vi "test_resist_new.vi"() -> ()   [LabVIEW 2015]
panel:
  out "String":string
  in  "Stop Button":bool
  in  "Open Button":bool
  out "Waveform Chart":dbl(graph)
  out "Voltage value":string
  in  "Refresh Button":bool
  in  "Close VI":bool
  in  "Run Test":bool
  out "error out":errorcluster[](array[cluster])
  in  "Measure time (s)":string="300"
  in  "Acquisition frequency (s)":string="1"
  in  "Precision":string="3"
  # "Insert measure parameters and then click \"Run test\""
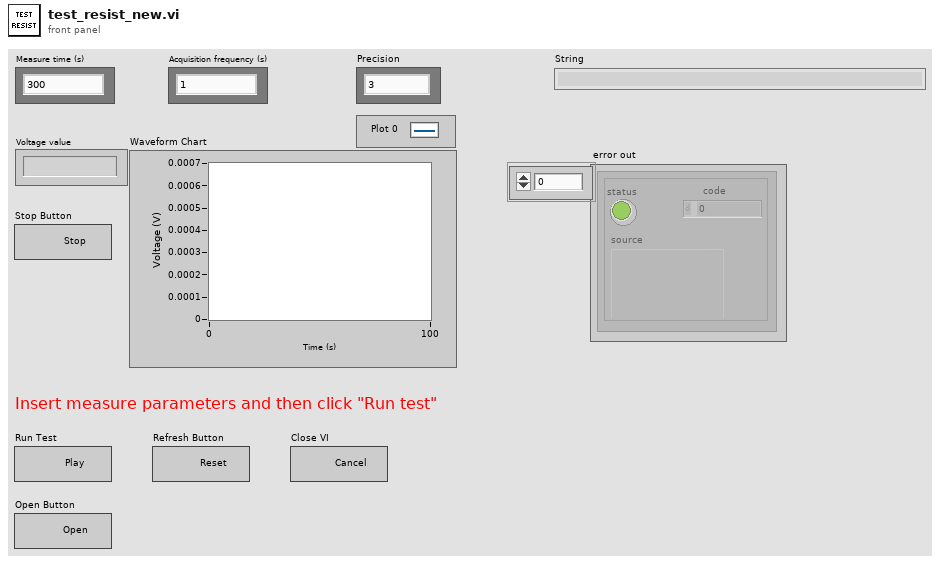
[diagram p1: front panel]
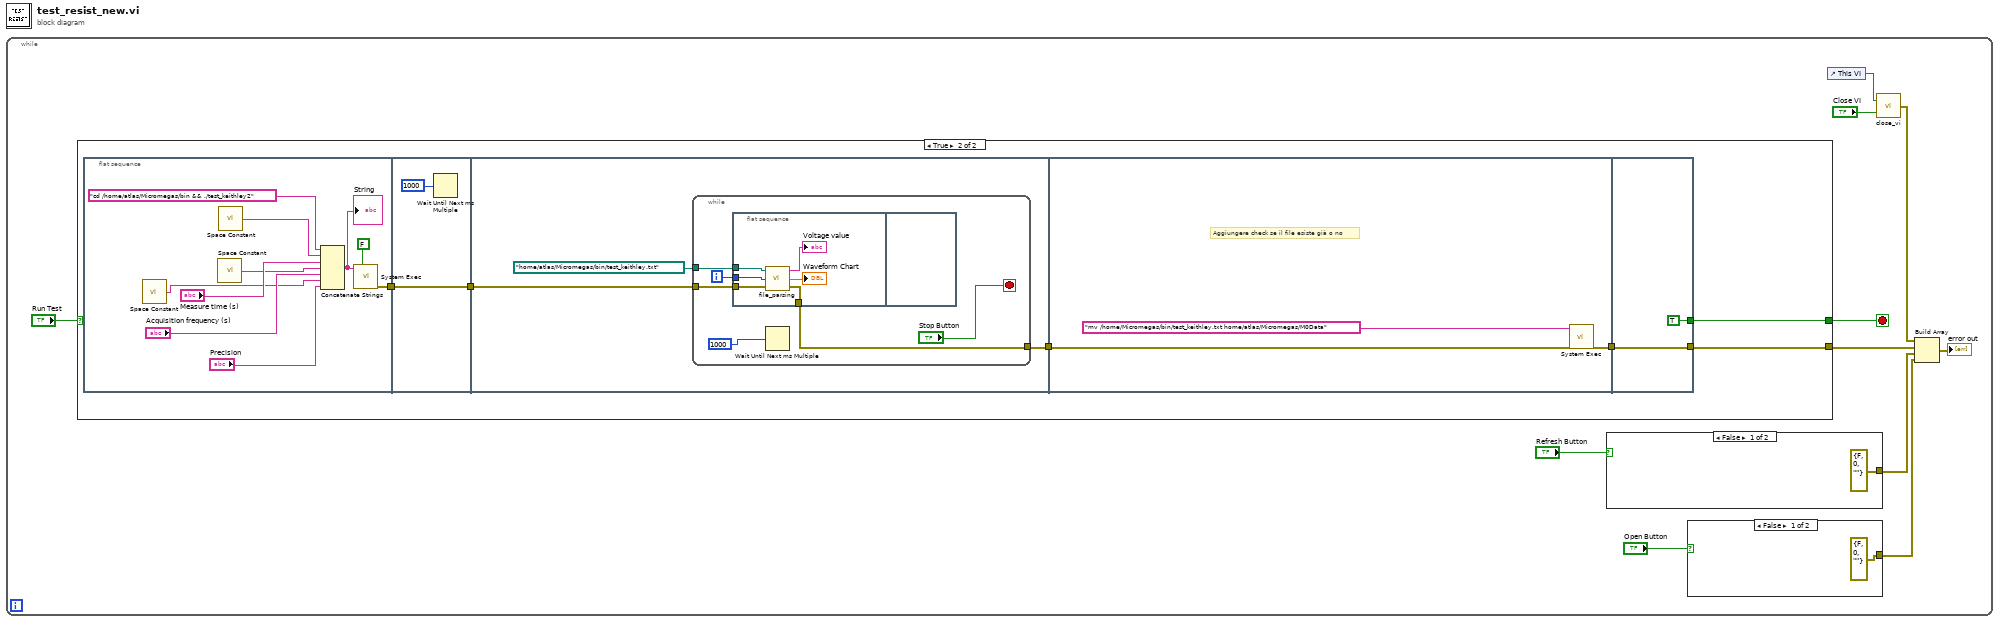
[diagram p0: block diagram]
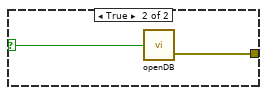
[diagram p2: hidden frame]
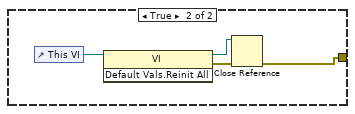
[diagram p3: hidden frame]
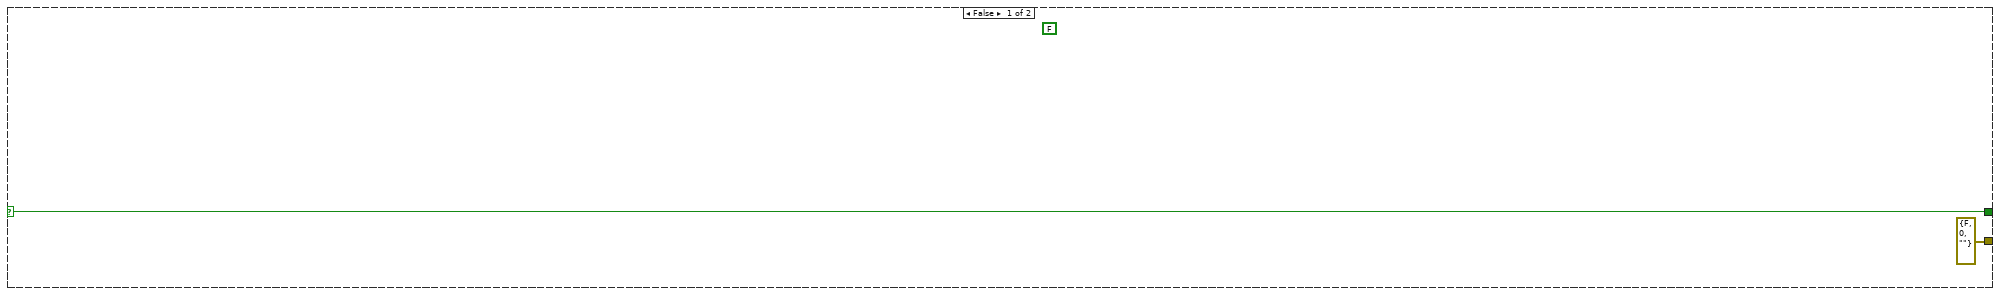
[diagram p4: hidden frame]
diagram:
  n1 = while {
    stop <- w1 stop-if-true
    n2 = case shown="True" "Run Test" {
      selector: "Run Test" -> [w21 _]
      tunnel: [w21 w25] -> w1
      tunnel: [errorcluster {"status"=FALSE, "code"=0, "source"=""} ("error out") w24] -> w8
      frame False {
        (unwired) FALSE
      }
      frame True {
        n3 = flat-sequence {
          tunnel: [w37] -> w23
          tunnel: w23 -> [w39]
          tunnel: [w39] -> w26
          tunnel: w26 -> [w42]
          tunnel: [w40] -> w22
          tunnel: [w56] -> w27
          tunnel: w22 -> [w55]
          tunnel: [TRUE] -> w25
          tunnel: [w58] -> w24
          tunnel: w27 -> [w58]
          frame #0 {
            n4 = call <vilib>:"Space Constant.vi"() -> ("String"=w31:string)
            n5 = call <vilib>:"Space Constant.vi"() -> ("String"=w33:string)
            n6 = call <vilib>:"Space Constant.vi"() -> ("String"=w35:string)
            n7 = Concatenate Strings("cd /home/atlas/Micromegas/bin && ./test_keithley2" ("String"), w35, "Measure time (s)", w33, "Acquisition frequency (s)", w31, "Precision") -> (w29:string)
            "String" <- w29
            n8 = call <vilib>:"System Exec.vi"("wait until completion? (T)"=FALSE, "command line"=w29) -> ("error out"=w37:errorcluster)  [unwired: 6 in, 3 out]
          }
          frame #1 {
            n9 = Wait Until Next ms Multiple(millisecond multiple=u32 1000) -> ()  [unwired: 1 out]
          }
          frame #2 {
            n10 = while {
              tunnel: w42 -> [w46]
              tunnel: path "/home/atlas/Micromegas/bin/test_keithley.txt" -> [w48]
              tunnel: [w45] -> w40
              i -> [w47]
              stop <- "Stop Button" stop-if-true
              n11 = flat-sequence {
                tunnel: w48 -> [w54]
                tunnel: w47 -> [w53]
                tunnel: w46 -> [w52]
                tunnel: [w49] -> w45
                frame #0 {
                  n12 = call "file_parsing.vi"("error in"=w52, "line index"=w53, "File Path Control"=w54) -> ("error out"=w49:errorcluster, "Waveform Chart"=→"Waveform Chart":dbl, "String"=→"Voltage value":string)
                }
                frame #1 {
                }
              }
              n13 = Wait Until Next ms Multiple(millisecond multiple=1000 ("y")) -> ()  [unwired: 1 out]
            }
          }
          frame #3 {
            # "Aggiungere check se il file esiste già o no"
            n14 = call <vilib>:"System Exec.vi"("error in (no error)"=w55, "command line"="mv /home/Micromegas/bin/test_keithley.txt home/atlas/Micromegas/M0Data") -> ("error out"=w56:errorcluster)  [unwired: 6 in, 3 out]
          }
          frame #4 {
          }
        }
      }
    }
    n15 = case shown="False" "Refresh Button" {
      tunnel: [errorcluster {"status"=FALSE, "code"=0, "source"=""} ("error out") w16] -> w7
      frame False {
      }
      frame True {
        n16 = control-ref of="This VI"() -> (w19:refnum<vi>)
        n17 = invoke class="VI" method="Default Vals.Reinit All"(reference=w19) -> (reference out=w18:refnum<vi>, error out=w17:errorcluster)  [unwired: 2 in, 1 out]
        n18 = Close Reference(reference=w18, error in (no error)=w17) -> (error out=w16:errorcluster)
      }
    }
    n19 = case shown="False" "Open Button" {
      selector: "Open Button" -> [_ w14]
      tunnel: [errorcluster {"status"=FALSE, "code"=0, "source"=""} ("error out") w13] -> w2
      frame False {
      }
      frame True {
        n20 = call "openDB.vi"("Open Button"=w14) -> ("error out"=w13:errorcluster)  [unwired: 1 out]
      }
    }
    n21 = control-ref of="This VI"() -> (w4:refnum<vi>)
    n22 = call "close_vi.vi"("Process Stop Button"="Close VI", "reference"=w4) -> ("error out"=w9:errorcluster)
    n23 = Build Array(w9, w8, w7, w2) -> (→"error out":errorcluster[])
  }
